vi "Write Persist State Enabled.vi"(8 "error in (no error)":errorcluster, 10 "Persist State Enabled":bool=TRUE, 11 "Rename in":refnum<class "Rename.lvclass">) -> (0 "error out":errorcluster, 3 "Rename out":refnum<class "Rename.lvclass">)   [LabVIEW 2015, in "Generic Module Library.lvlib" / "Template G_Module.lvlib" / "Rename.lvclass"]
uses:
  Rename.lvclass
  Rename.lvclass/Rename.ctl
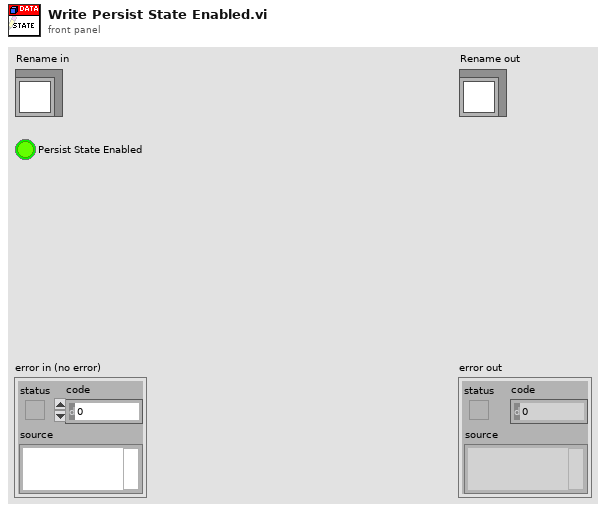
[diagram p1: front panel]
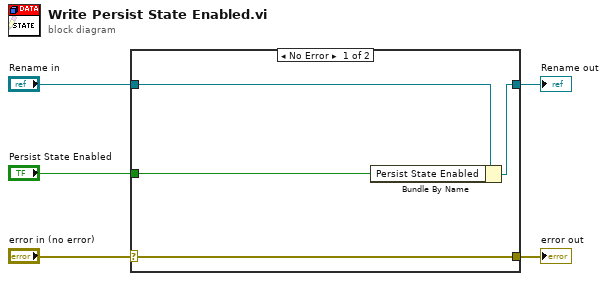
[diagram p0: block diagram]
diagram:
  n1 = case shown="No Error" "error in (no error)" {
    selector: "error in (no error)" -> [w9 w10]
    tunnel: [w9 w10] -> w4
    tunnel: [w7 w11] -> w2
    tunnel: "Rename in" -> [w8 w11]
    tunnel: "Persist State Enabled" -> [w6 _]
    frame No Error {
      n2 = Bundle By Name(cluster=w8, "Persist State Enabled"=w6) -> (w7:refnum<class "Rename.lvclass">)
    }
    frame Error {
    }
  }
  "error out" <- w4
  "Rename out" <- w2
